vi "Test reading 5052 and writing to database.vi"   [LabVIEW 2017]
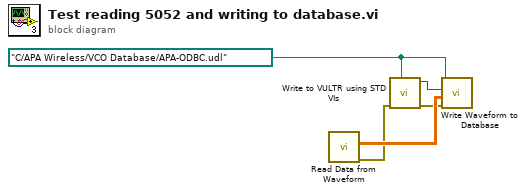
[diagram p0: block diagram]
diagram:
  w5 = path "C:/APA Wireless/VCO Database/APA-ODBC.udl" ("conninfo")
  n1 = call "Read Data from  Waveform.vi"() -> ("error out"=w3:errorcluster, "Results"=w4:sgl[][])  [unwired: 10 in]
  n2 = call "Write to VULTR using STD VIs.vi"("conninfo"=w5, "error in (no error)"=w3) -> ("error out"=w2:errorcluster, "Get FrequencyID"=w1:i32)  [unwired: 8 in]
  n3 = call "Write Waveform to Database.vi"("error in (no error)"=w2, "Array"=w4, "FreqID"=w1, "conninfo"=w5) -> ()  [unwired: 7 in, 1 out]
